vi "Parse Tags.vi"(11 "Tags":string) -> (3 "Tags":string[](array[string]))   [LabVIEW 2017, in "Feed.lvclass"]
uses:
  <vilib>/NI_RSS/Feed/Feed.lvclass
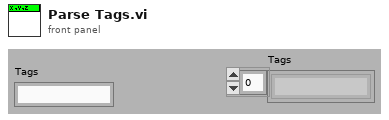
[diagram p1: front panel]
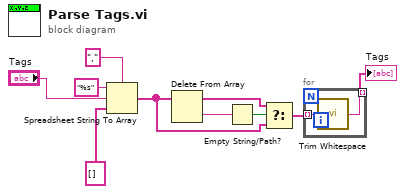
[diagram p0: block diagram]
diagram:
  n1 = Spreadsheet String To Array(delimiter (Tab)=",", format string="%s", spreadsheet string="Tags", array type (2D Dbl)=string[] []) -> (array=w3:string[])
  n2 = Delete From Array(array=w3) -> (deleted portion=w6:string, array with subset deleted=w4:string[])  [unwired: 2 in]
  n3 = Empty String/Path?(string/path=w6) -> (empty?=w5:bool)
  n4 = Select(t=w4, s=w5, f=w3) -> (s? t:f=w2:string[])
  n5 = for {
    tunnel: w2 -> [w12] mode=indexing
    tunnel: [w11] -> w1 mode=indexing
    n6 = call <vilib>:"Trim Whitespace.vi"("string"=w12) -> ("trimmed string"=w11:string)  [unwired: 1 in]
  }
  "Tags" <- w1
